vi "LV to ITX Retrieve SM.vi"(0 "File or Folder Path":path=path "C:/", 1 "Data Type":T3=enum."DAT", 2 "DAT header length":i32=11, 5 "offset":i32, 7 "length":i32=1, 11 "error in (no error)":errorcluster) -> (4 "A vs B":cluster{dbl[], dbl[]}[](graph), 6 "C vs D":cluster{dbl[], dbl[]}[](graph), 8 "E":dbl[][](graph), 14 "Notes":string)   [LabVIEW 2019, in "LV-Data.ITX.lvclass"]
uses:
  LV-Data.ITX.lvclass
  <vilib>/Utility/miscctls.llb/LVOffsetAndMultiplierTypeDef.ctl
  Typedefs/Retrieve Data Type.ctl
  LV-Data/Typedefs/Map Variant--map.ctl
  b9190c8c-04b9-4fe6-9890-9f3313ef96ba.vi
  59021a08-4f23-4d52-b62b-93f2ba281558.vi
  LV-Data/LV-Data.lvclass
  <userlib>/LevyLab/Graph Utilities/graph_utilities.lvclass
  <userlib>/LevyLab/Instrument Framework/SMOs/Instrument/Instrument.lvclass
panel:
  out "Current State":string
  in  "Update Graphs":bool
  in  "Read Files":bool
  in  "Initialize Keys":bool
  out "N":T1(array[cluster]) {"N5" format="%#_6p"; "N4" format="%#_6p"; "N3" format="%#_6p"; "N2" format="%#_6p"; "N1" format="%#_6p"}
  in  "keys":T2 {"N5" items=["AI1", "AI10", "AI11", "AI12", "AI2", "AI3", "AI4", "AI5", "AI6", "AI7", "AI8", "AI9", "AO1", "AO10", "AO11", "AO12", "AO2", "AO3", "AO4", "AO5", "AO6", "AO7", "AO8", "AO9", "Magnet", "Magnet Field", "OFF", "Temperature", "Time", "X1", "X10", "X11", "X12", "X2", "X3", "X4", "X5", "X6", "X7", "X8", "X9", "Y1", "Y10", "Y11", "Y12", "Y2", "Y3", "Y4", "Y5", "Y6", "Y7", "Y8", "Y9"]; "N4" items=["AI1", "AI10", "AI11", "AI12", "AI2", "AI3", "AI4", "AI5", "AI6", "AI7", "AI8", "AI9", "AO1", "AO10", "AO11", "AO12", "AO2", "AO3", "AO4", "AO5", "AO6", "AO7", "AO8", "AO9", "Magnet", "Magnet Field", "OFF", "Temperature", "Time", "X1", "X10", "X11", "X12", "X2", "X3", "X4", "X5", "X6", "X7", "X8", "X9", "Y1", "Y10", "Y11", "Y12", "Y2", "Y3", "Y4", "Y5", "Y6", "Y7", "Y8", "Y9"]; "N3" items=["AI1", "AI10", "AI11", "AI12", "AI2", "AI3", "AI4", "AI5", "AI6", "AI7", "AI8", "AI9", "AO1", "AO10", "AO11", "AO12", "AO2", "AO3", "AO4", "AO5", "AO6", "AO7", "AO8", "AO9", "Magnet", "Magnet Field", "OFF", "Temperature", "Time", "X1", "X10", "X11", "X12", "X2", "X3", "X4", "X5", "X6", "X7", "X8", "X9", "Y1", "Y10", "Y11", "Y12", "Y2", "Y3", "Y4", "Y5", "Y6", "Y7", "Y8", "Y9"]; "N2" items=["AI1", "AI10", "AI11", "AI12", "AI2", "AI3", "AI4", "AI5", "AI6", "AI7", "AI8", "AI9", "AO1", "AO10", "AO11", "AO12", "AO2", "AO3", "AO4", "AO5", "AO6", "AO7", "AO8", "AO9", "Magnet", "Magnet Field", "OFF", "Temperature", "Time", "X1", "X10", "X11", "X12", "X2", "X3", "X4", "X5", "X6", "X7", "X8", "X9", "Y1", "Y10", "Y11", "Y12", "Y2", "Y3", "Y4", "Y5", "Y6", "Y7", "Y8", "Y9"]; "N1" items=["AI1", "AI10", "AI11", "AI12", "AI2", "AI3", "AI4", "AI5", "AI6", "AI7", "AI8", "AI9", "AO1", "AO10", "AO11", "AO12", "AO2", "AO3", "AO4", "AO5", "AO6", "AO7", "AO8", "AO9", "Magnet", "Magnet Field", "OFF", "Temperature", "Time", "X1", "X10", "X11", "X12", "X2", "X3", "X4", "X5", "X6", "X7", "X8", "X9", "Y1", "Y10", "Y11", "Y12", "Y2", "Y3", "Y4", "Y5", "Y6", "Y7", "Y8", "Y9"]; "E" items=["AI1", "AI10", "AI11", "AI12", "AI2", "AI3", "AI4", "AI5", "AI6", "AI7", "AI8", "AI9", "AO1", "AO10", "AO11", "AO12", "AO2", "AO3", "AO4", "AO5", "AO6", "AO7", "AO8", "AO9", "Magnet", "Magnet Field", "OFF", "Temperature", "Time", "X1", "X10", "X11", "X12", "X2", "X3", "X4", "X5", "X6", "X7", "X8", "X9", "Y1", "Y10", "Y11", "Y12", "Y2", "Y3", "Y4", "Y5", "Y6", "Y7", "Y8", "Y9"]; "D" items=["AI1", "AI10", "AI11", "AI12", "AI2", "AI3", "AI4", "AI5", "AI6", "AI7", "AI8", "AI9", "AO1", "AO10", "AO11", "AO12", "AO2", "AO3", "AO4", "AO5", "AO6", "AO7", "AO8", "AO9", "Magnet", "Magnet Field", "OFF", "Temperature", "Time", "X1", "X10", "X11", "X12", "X2", "X3", "X4", "X5", "X6", "X7", "X8", "X9", "Y1", "Y10", "Y11", "Y12", "Y2", "Y3", "Y4", "Y5", "Y6", "Y7", "Y8", "Y9"]; "C" items=["AI1", "AI10", "AI11", "AI12", "AI2", "AI3", "AI4", "AI5", "AI6", "AI7", "AI8", "AI9", "AO1", "AO10", "AO11", "AO12", "AO2", "AO3", "AO4", "AO5", "AO6", "AO7", "AO8", "AO9", "Magnet", "Magnet Field", "OFF", "Temperature", "Time", "X1", "X10", "X11", "X12", "X2", "X3", "X4", "X5", "X6", "X7", "X8", "X9", "Y1", "Y10", "Y11", "Y12", "Y2", "Y3", "Y4", "Y5", "Y6", "Y7", "Y8", "Y9"]; "B" items=["AI1", "AI10", "AI11", "AI12", "AI2", "AI3", "AI4", "AI5", "AI6", "AI7", "AI8", "AI9", "AO1", "AO10", "AO11", "AO12", "AO2", "AO3", "AO4", "AO5", "AO6", "AO7", "AO8", "AO9", "Magnet", "Magnet Field", "OFF", "Temperature", "Time", "X1", "X10", "X11", "X12", "X2", "X3", "X4", "X5", "X6", "X7", "X8", "X9", "Y1", "Y10", "Y11", "Y12", "Y2", "Y3", "Y4", "Y5", "Y6", "Y7", "Y8", "Y9"]; "A" items=["AI1", "AI10", "AI11", "AI12", "AI2", "AI3", "AI4", "AI5", "AI6", "AI7", "AI8", "AI9", "AO1", "AO10", "AO11", "AO12", "AO2", "AO3", "AO4", "AO5", "AO6", "AO7", "AO8", "AO9", "Magnet", "Magnet Field", "OFF", "Temperature", "Time", "X1", "X10", "X11", "X12", "X2", "X3", "X4", "X5", "X6", "X7", "X8", "X9", "Y1", "Y10", "Y11", "Y12", "Y2", "Y3", "Y4", "Y5", "Y6", "Y7", "Y8", "Y9"]}
  in  "OK":bool
  in  "D  is time?":bool
  in  "B is time?":bool
  out "time":string[][](table)
  in  "Use Folder Index File?":bool
  in  "Generate Folder Index File?":bool
  in  "Ez name":string="Ez name"
  in  "Ey name":string="Ey name"
  in  "Ex name":string="Ex name"
  in  "C y name":string="C y name"
  in  "D x name":string="D x name"
  in  "A y name":string="A y name"
  in  "B x name":string="B x name"
  out "Index, Wavenames":string[][](table)
  in  "recolor traces?":bool
  in  "Ex":T4={"Offset"=0.0, "Multiplier"=1.0}
  in  "Ey":T4={"Offset"=0.0, "Multiplier"=1.0}
  out "counter":i32
  out "pattern":string="*.dat"
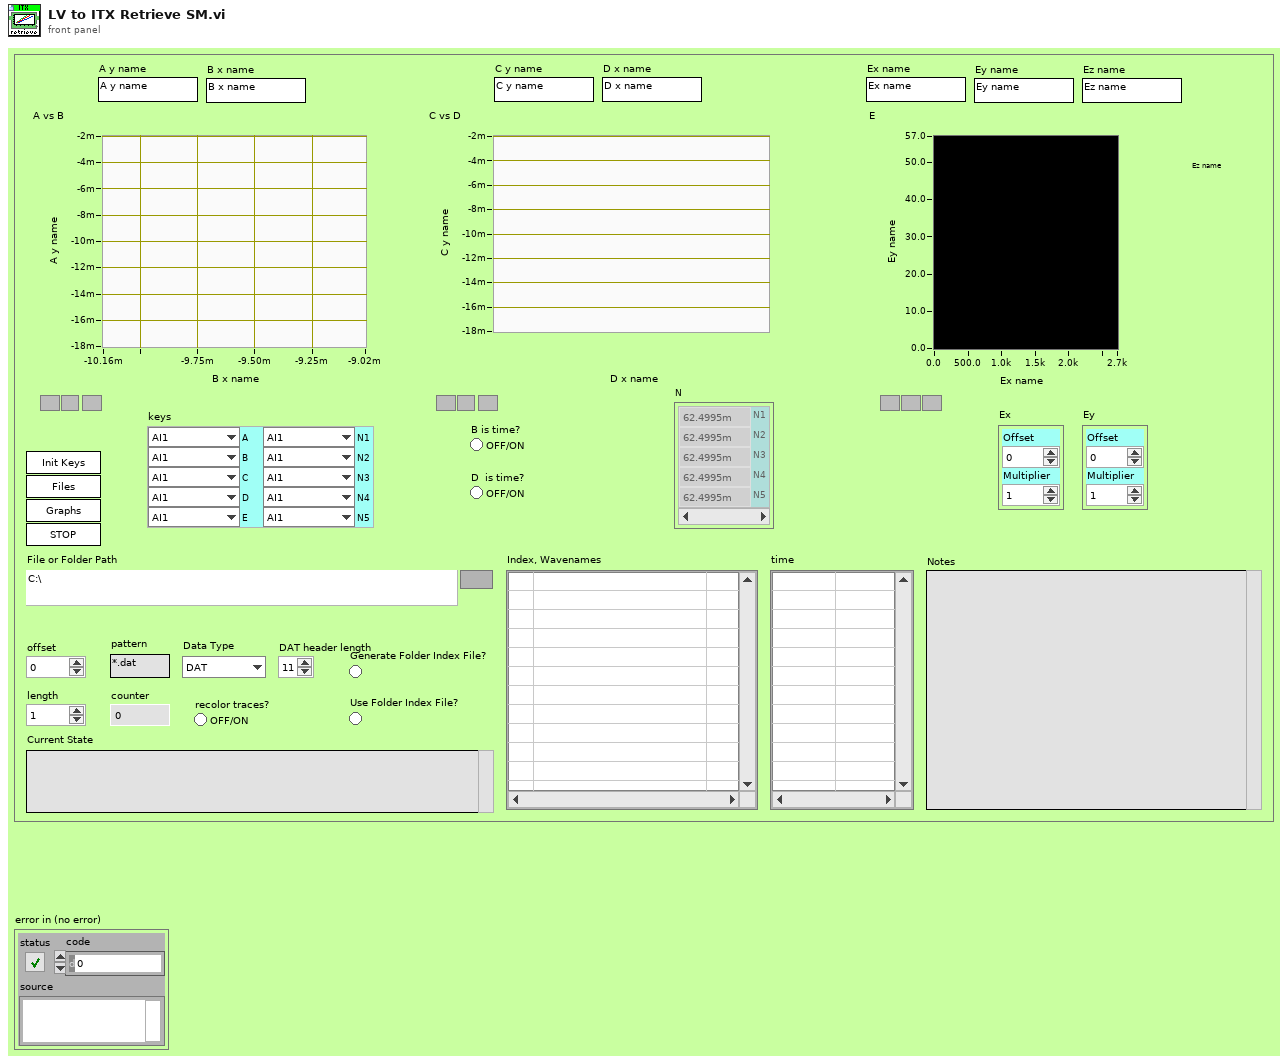
[diagram p1: front panel]
types:
  T1 = cluster{"N1":dbl, "N2":dbl, "N3":dbl, "N4":dbl, "N5":dbl}[]
  T2 = cluster{"A":u16, "B":u16, "C":u16, "D":u16, "E":u16, "N1":u16, "N2":u16, "N3":u16, "N4":u16, "N5":u16}
  T3 = typedef "LV-Data.ITX.lvclass/Retrieve Data Type.ctl" = enum16{"ITX", "ITX w/ 2D", "DAT", "TDMS"}
  T4 = typedef "LVOffsetAndMultiplierTypeDef.ctl" = cluster{"Offset":dbl, "Multiplier":dbl}
  T5 = enum32{"Invalid", "Standard", "Closed", "Hidden", "Minimized", "Maximized"}
  T6 = enum32{"invalid app kind", "Development System", "Run Time System", "Student Edition", "Embedded LabVIEW", "Evaluation", "Custom"}
  T7 = typedef "LV-Data.lvclass/Map Variant--map.ctl" = map{string, variant}
  T8 = cluster{"N1":dbl, "N2":dbl, "N3":dbl, "N4":dbl, "N5":dbl}
  T9 = cluster{"Core":cluster{"Current VI Reference":refnum<vi>, "Close Panel on Exit?":bool}, "Files":path[], "Append Index":i32, "Running Step":i32, "Data Map":T7[], "ring map":map{string, refnum<vi>}, "Wavenames":string[], "A vs B":cluster{dbl[], dbl[]}[], "C vs D":cluster{dbl[], dbl[]}[], "E":dbl[][]}
  T10 = cluster{"Current VI Reference":refnum<vi>, "Close Panel on Exit?":bool}
  T11 = typedef "LV-Data.lvclass/Dictionary--cluster.ctl" = cluster{"key":string, "value":variant}
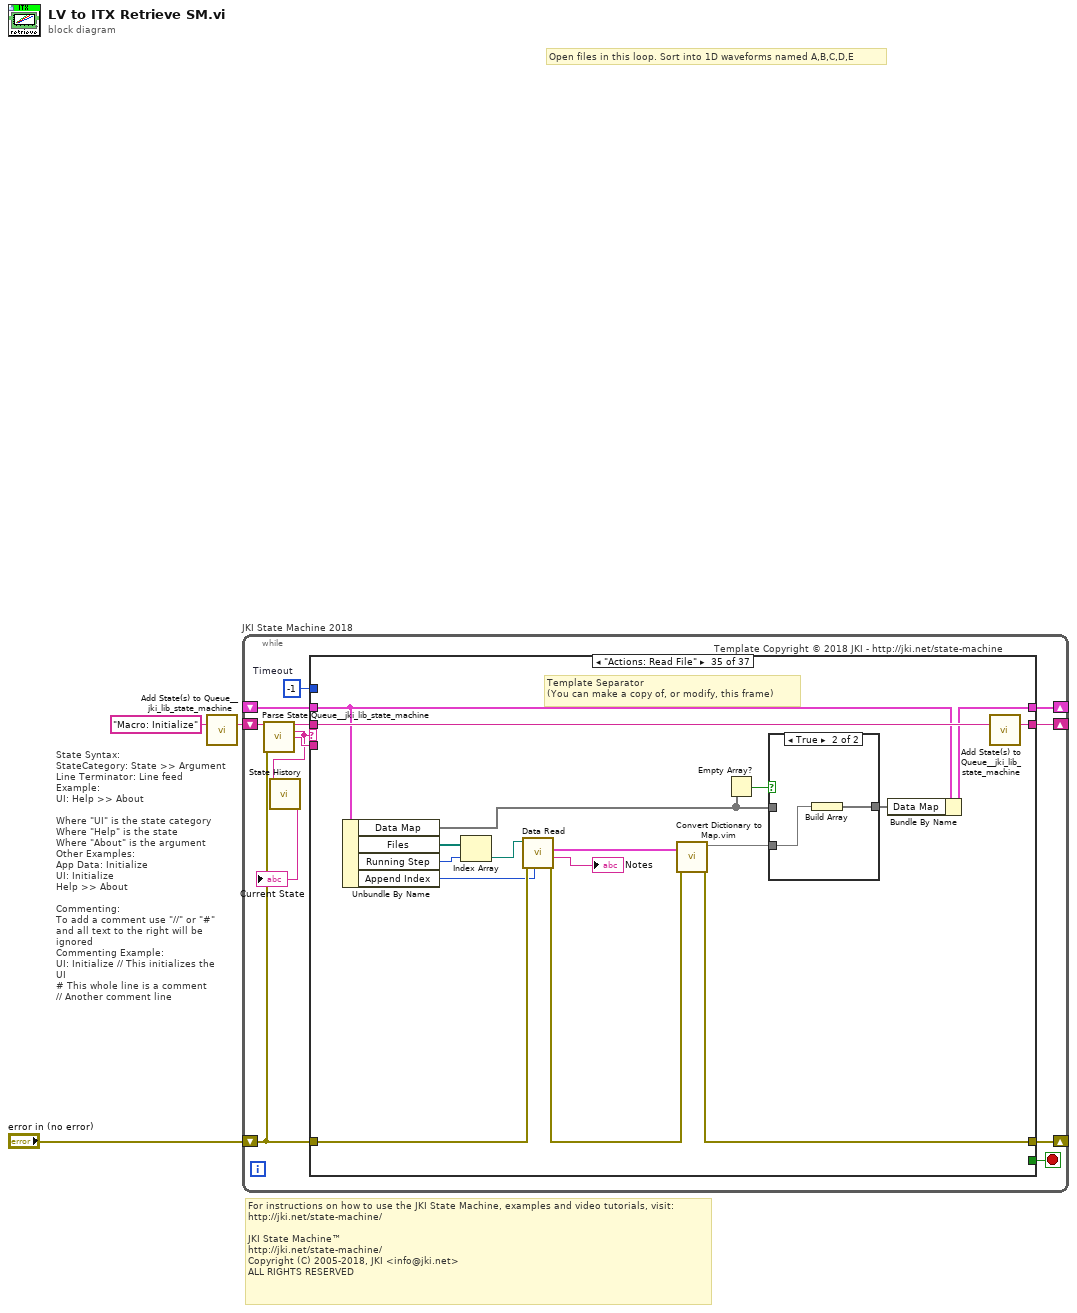
[diagram p0: block diagram]
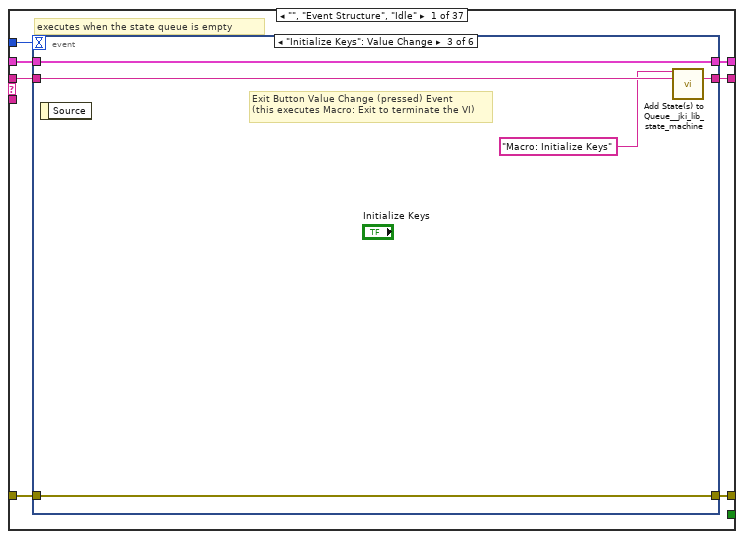
[diagram p2: hidden frame]
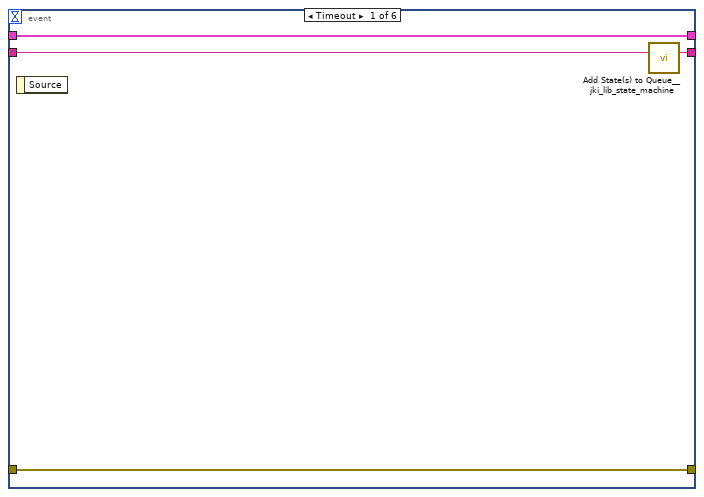
[diagram p3: hidden frame]
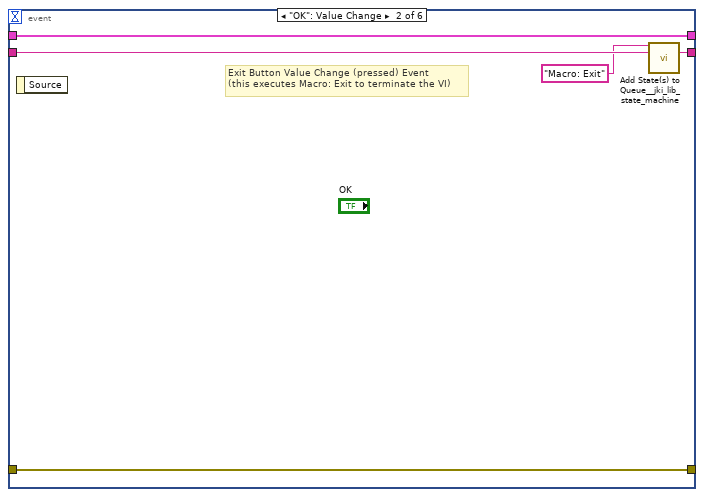
[diagram p4: hidden frame]
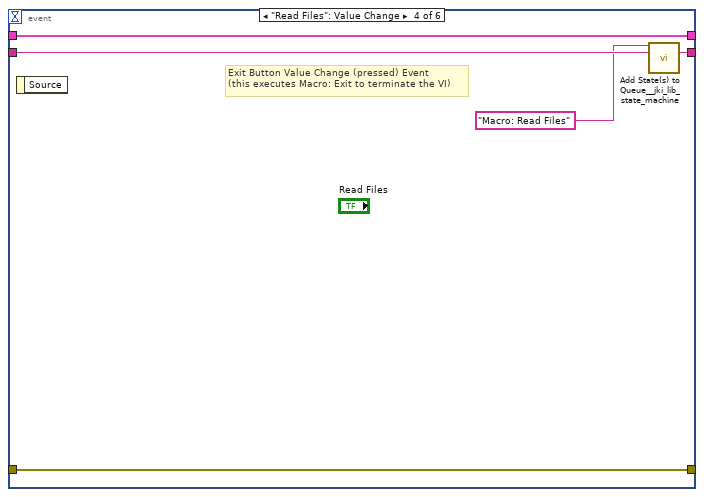
[diagram p5: hidden frame]
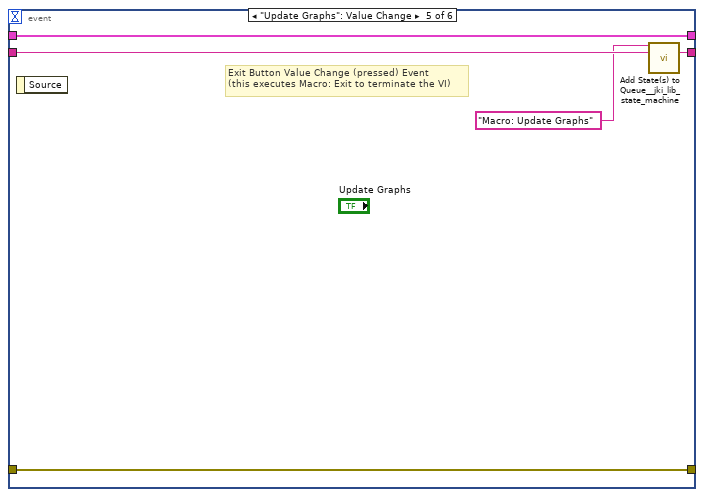
[diagram p6: hidden frame]
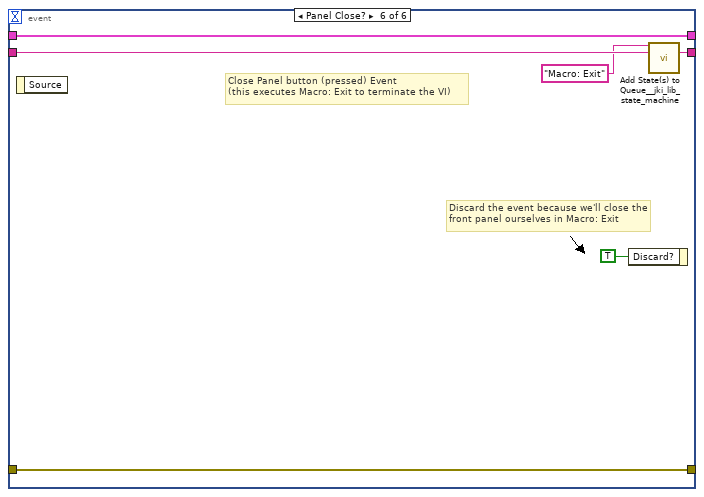
[diagram p7: hidden frame]
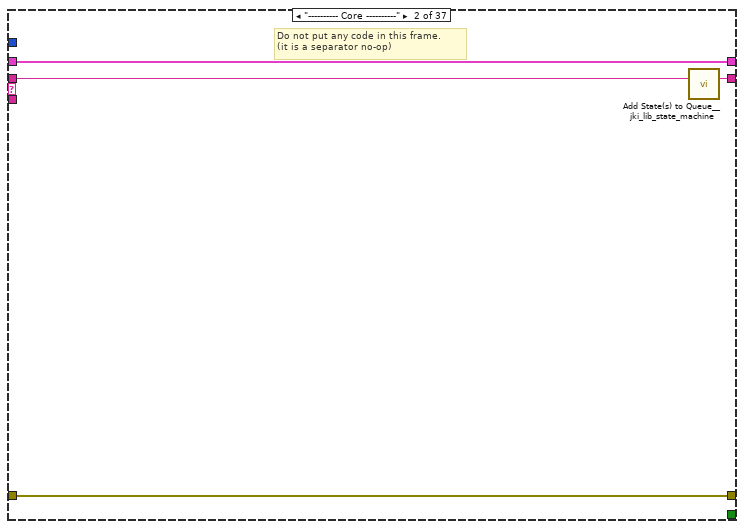
[diagram p8: hidden frame]
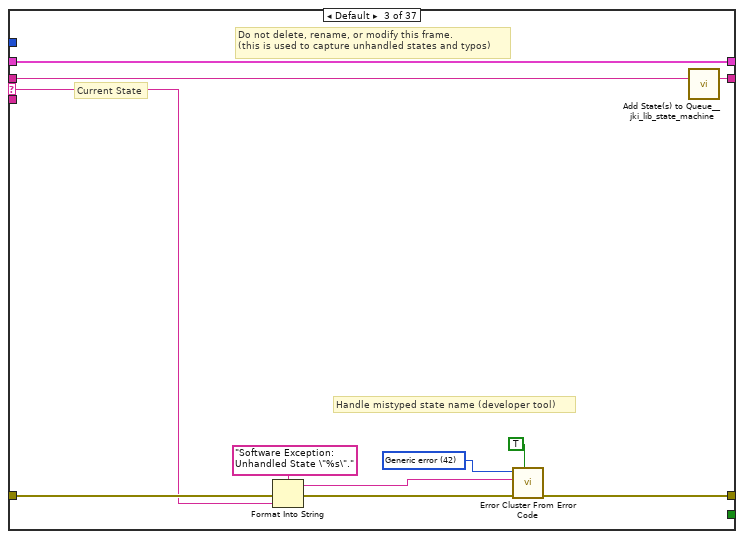
[diagram p9: hidden frame]
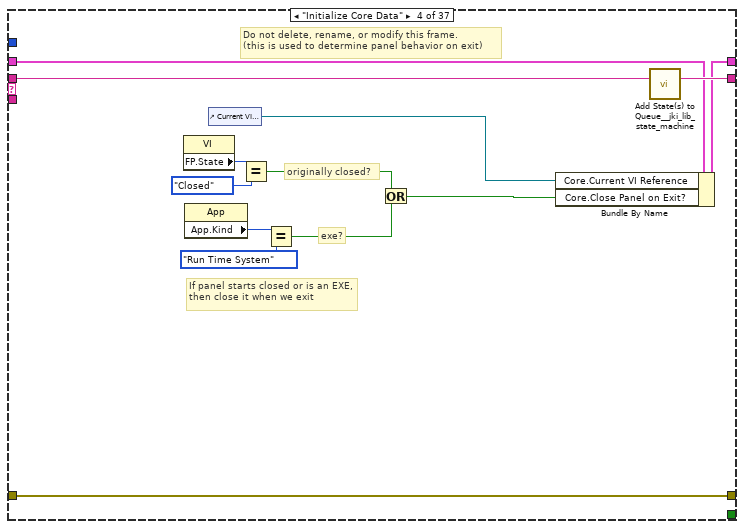
[diagram p10: hidden frame]
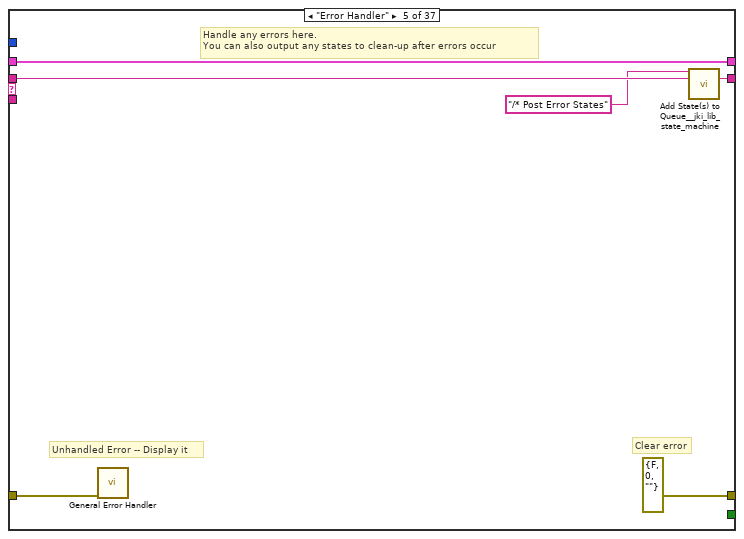
[diagram p11: hidden frame]
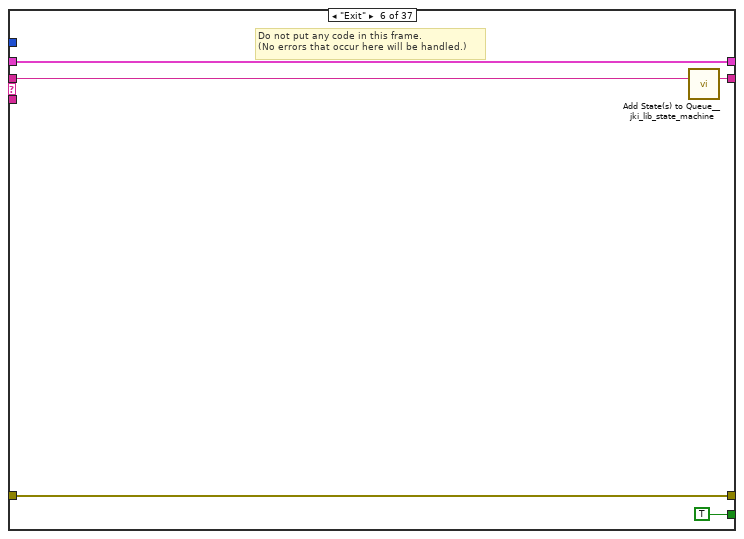
[diagram p12: hidden frame]
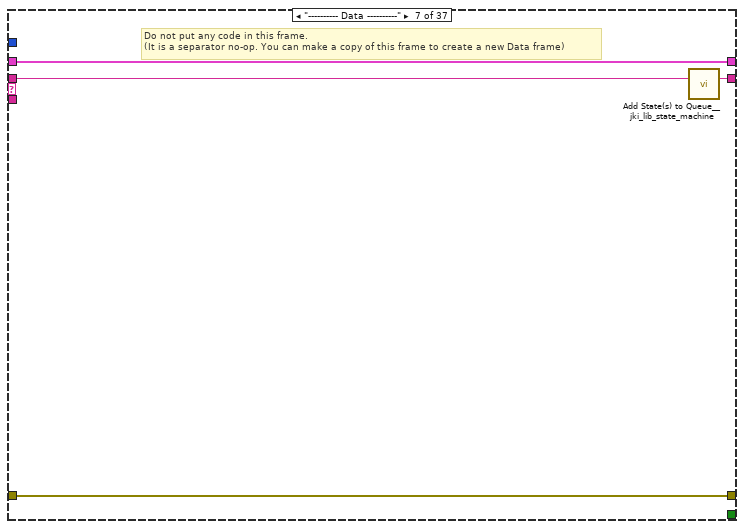
[diagram p13: hidden frame]
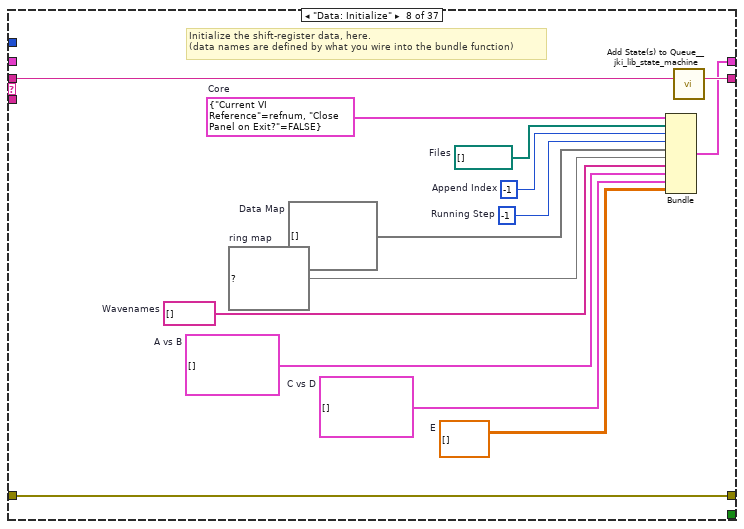
[diagram p14: hidden frame]
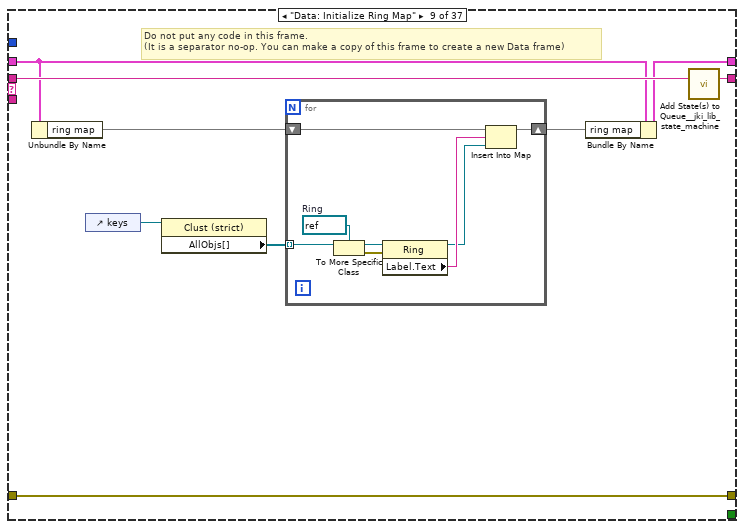
[diagram p15: hidden frame]
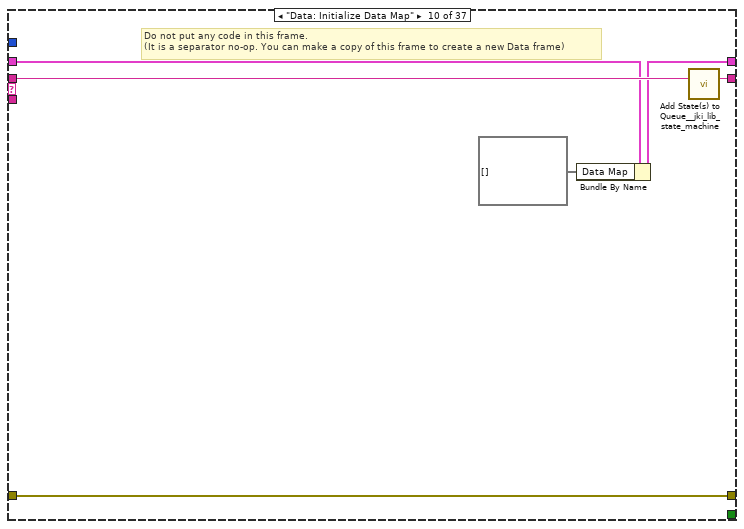
[diagram p16: hidden frame]
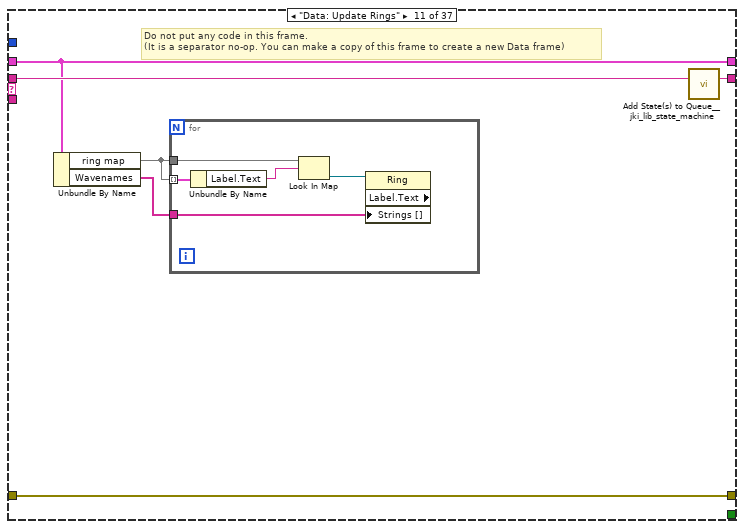
[diagram p17: hidden frame]
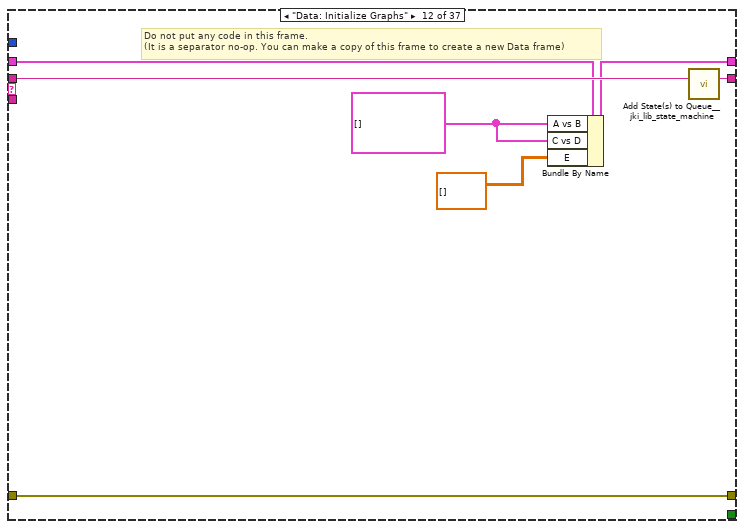
[diagram p18: hidden frame]
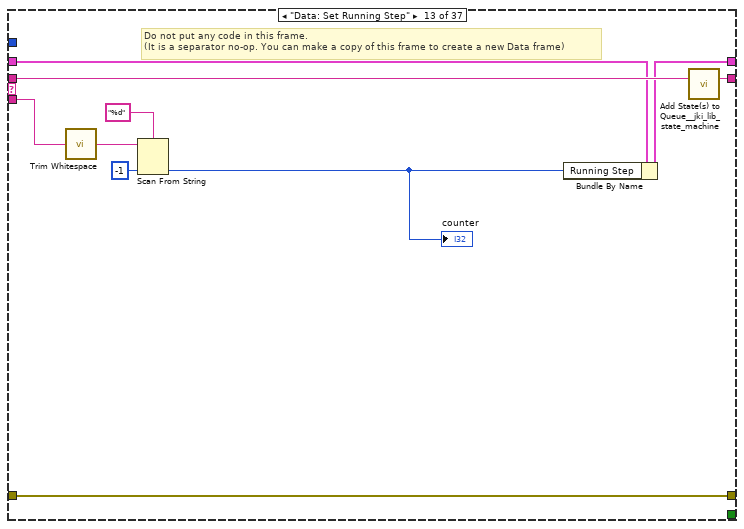
[diagram p19: hidden frame]
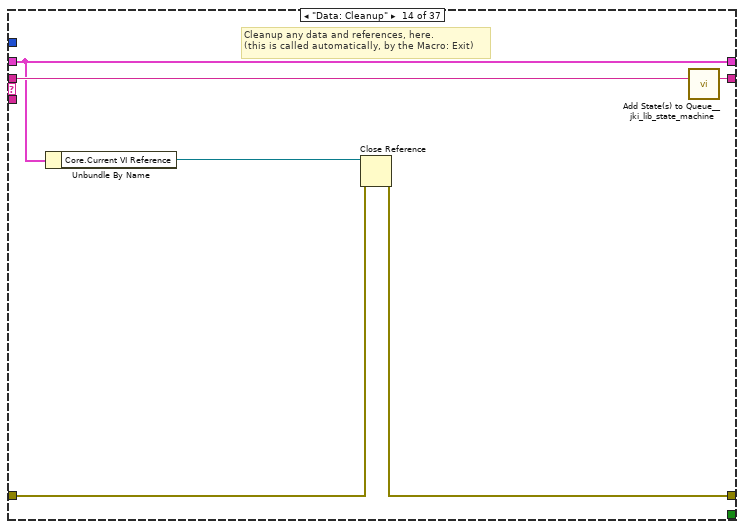
[diagram p20: hidden frame]
diagram:
  # "For instructions on how to use the JKI State Machine, examples and video tutorials, visit:\nhttp://jki.net/state-machine/\n\nJKI State Machine™\nhttp://jki.net/state-machine/\nCopyright (C) 2005-2018, JKI <info@jki.net>\nALL RIGHTS RESERVED"
  # "State Syntax:\nStateCategory: State >> Argument\nLine Terminator: Line feed\nExample:\nUI: Help >> About\n\nWhere \"UI\" is the state category\nWhere \"Help\" is the state\nWhere \"About\" is the argument\nOther Examples:\nApp Data: Initialize\nUI: Initialize\nHelp >> About\n\nCommenting:\nTo add a comment use \"//\" or \"#\" and all text to the right will be ignored\nCommenting Example:\nUI: Initialize // This initializes the UI\n# This whole line is a comment\n// Another comment line"
  # "Open files in this loop. Sort into 1D waveforms named A,B,C,D,E"
  n1 = call <vilib>:"Add State(s) to Queue__jki_lib_state_machine.vi"("State(s) in (\"\")"="Macro: Initialize") -> ("States Out"=w3:string)  [unwired: 14 in]
  n2 = while "JKI State Machine 2018" {
    shift-right: [w9] -> _
    shift-left: _ -> [w8]
    shift-right: [w12] -> _
    shift-left: "error in (no error)" -> [w6]
    shift-right: [w11] -> _
    shift-left: w3 -> [w13]
    stop <- w10 stop-if-true
    w7 = -1  # Timeout
    # "Template Copyright © 2018 JKI - http://jki.net/state-machine"
    n3 = call <vilib>:"Parse State Queue__jki_lib_state_machine.vi"("State Queue"=w13, "Error In (no error)"=w6) -> ("Remaining States"=w15:string, "Current State"=w5:string, "Arguments"=w14:string)  [unwired: 11 in]
    n4 = call <userlib>:"State History.vi"("Current State"=w5) -> ("History"=→"Current State":string)  [unwired: 10 in]
    n5 = case shown="\"Actions: Read File\"" w5 {
      selector: w5 -> [_ _ w57 _ _ _ _ _ _ _ _ _ _ _ _ _ _ _ _ _ _ _ _ _ _ _ _ _ _ _ _ _ _ _ _ _ _]
      tunnel: w15 -> [w22 w56 w61 w80 w86 w91 w95 w109 w118 w132 w138 w150 w160 w166 w170 w176 w182 w194 w200 w228 w235 w304 w309 w314 w329 w334 w339 w344 w349 w359 w363 w377 w424 w446 w465 w499 w520]
      tunnel: w14 -> [_ _ _ _ _ _ _ _ _ _ _ _ w155 _ _ _ w177 _ _ _ w229 _ _ _ w319 _ _ _ _ _ _ _ _ _ _ _ _]
      tunnel: w8 -> [w20 w53 w59 w73 w83 w89 w92 _ w110 w128 w135 w146 w156 w161 w167 w174 w180 w191 w196 w225 w231 w301 w306 w311 w326 w331 w336 w341 w346 w356 w360 w366 w419 w439 w454 w471 w517]
      tunnel: [w19 w54 w63 w77 errorcluster {"status"=FALSE, "code"=0, "source"=""} ("error out") w88 w93 w106 w116 w130 w136 w148 w158 w162 w168 w172 w178 w192 w198 w226 w232 w302 w307 w312 w327 w332 w337 w342 w347 w357 w361 w370 w422 w442 w456 w497 w518] -> w12
      tunnel: w6 -> [w18 w54 w62 w77 w82 w88 w93 w106 w116 w130 w136 w148 w158 w163 w168 w171 w179 w192 w198 w226 w233 w302 w307 w312 w327 w332 w337 w342 w347 w357 w361 w369 w422 w441 w461 w497 w518]
      tunnel: [w21 w55 w60 w79 w85 w90 w94 w108 w117 w131 w137 w149 w159 w165 w169 w175 w181 w193 w199 w227 w234 w303 w308 w313 w328 w333 w338 w343 w348 w358 w362 w376 w423 w445 w464 w498 w519] -> w11
      tunnel: [_ _ _ _ _ TRUE _ _ _ _ _ _ _ _ _ _ _ _ _ _ _ _ _ _ _ _ _ _ _ _ _ _ _ _ _ _ _] -> w10
      tunnel: [w17 w53 w59 w78 w83 w89 w92 w107 w111 w129 w135 w147 w157 w161 w167 w174 w180 w191 w196 w225 w231 w301 w306 w311 w326 w331 w336 w341 w346 w356 w360 w367 w420 w440 w455 w472 w517] -> w9
      tunnel: w7 -> [w16 _ _ _ _ _ _ _ _ _ _ _ _ _ _ _ _ _ _ _ _ _ _ _ _ _ _ _ _ _ _ _ _ _ _ _ _]
      frame "", "Event Structure", "Idle" {
        # "executes when the state queue is empty"
        n6 = event shown="[2] \"Initialize Keys\": Value Change" {
          selector: _ -> [_ _ _ _ _ _]
          dyn-events: _ -> [_ _ _ _ _ _]
          timeout: w16 -> [_ _ _ _ _ _]
          tunnel: w22 -> [w26 w31 w36 w41 w46 w52]
          tunnel: [w25 w30 w35 w40 w45 w51] -> w21
          tunnel: w20 -> [w23 w28 w33 w38 w43 w49]
          tunnel: [w24 w29 w34 w39 w44 w50] -> w19
          tunnel: w18 -> [w24 w29 w34 w39 w44 w50]
          tunnel: [w23 w28 w33 w38 w43 w49] -> w17
          event Timeout {
            n7 = event-data() -> ()  [unwired: 1 in, 1 out]
            n8 = call <vilib>:"Add State(s) to Queue__jki_lib_state_machine.vi"("State(s) in (\"\")"=w26) -> ("States Out"=w25:string)  [unwired: 14 in]
          }
          event "OK": Value Change {
            # "Exit Button Value Change (pressed) Event\n(this executes Macro: Exit to terminate the VI)"
            n9 = event-data() -> ()  [unwired: 1 in, 1 out]
            n10 = call <vilib>:"Add State(s) to Queue__jki_lib_state_machine.vi"("State(s) in Front (\"\")"="Macro: Exit", "State(s) in (\"\")"=w31) -> ("States Out"=w30:string)  [unwired: 13 in]
          }
          event "Initialize Keys": Value Change {
            # "Exit Button Value Change (pressed) Event\n(this executes Macro: Exit to terminate the VI)"
            n11 = event-data() -> ()  [unwired: 1 in, 1 out]
            n12 = call <vilib>:"Add State(s) to Queue__jki_lib_state_machine.vi"("State(s) in Front (\"\")"="Macro: Initialize Keys", "State(s) in (\"\")"=w36) -> ("States Out"=w35:string)  [unwired: 13 in]
          }
          event "Read Files": Value Change {
            # "Exit Button Value Change (pressed) Event\n(this executes Macro: Exit to terminate the VI)"
            n13 = event-data() -> ()  [unwired: 1 in, 1 out]
            n14 = call <vilib>:"Add State(s) to Queue__jki_lib_state_machine.vi"("State(s) in Front (\"\")"="Macro: Read Files", "State(s) in (\"\")"=w41) -> ("States Out"=w40:string)  [unwired: 13 in]
          }
          event "Update Graphs": Value Change {
            # "Exit Button Value Change (pressed) Event\n(this executes Macro: Exit to terminate the VI)"
            n15 = event-data() -> ()  [unwired: 1 in, 1 out]
            n16 = call <vilib>:"Add State(s) to Queue__jki_lib_state_machine.vi"("State(s) in Front (\"\")"="Macro: Update Graphs", "State(s) in (\"\")"=w46) -> ("States Out"=w45:string)  [unwired: 13 in]
          }
          event Panel Close? {
            # "Discard the event because we'll close the front panel ourselves in Macro: Exit"
            # "Close Panel button (pressed) Event\n(this executes Macro: Exit to terminate the VI)"
            n17 = event-data() -> ()  [unwired: 1 in, 1 out]
            n18 = event-data("Discard?"=TRUE) -> ()  [unwired: 1 in, 1 out]
            n19 = call <vilib>:"Add State(s) to Queue__jki_lib_state_machine.vi"("State(s) in Front (\"\")"="Macro: Exit", "State(s) in (\"\")"=w52) -> ("States Out"=w51:string)  [unwired: 13 in]
          }
        }
      }
      frame "---------- Core ----------" {
        # "Do not put any code in this frame.\n(it is a separator no-op)"
        n20 = call <vilib>:"Add State(s) to Queue__jki_lib_state_machine.vi"("State(s) in (\"\")"=w56) -> ("States Out"=w55:string)  [unwired: 14 in]
      }
      frame Default {
        w66 = 42 items=["No error", "Argument error", "Memory is full", "Out of zone", "End of file", "File already open", "Generic file I/O error", "File not found", "File permission error", "Disk is full", "Duplicate path", "Too many files open", "System feature not enabled", "Resource file not found", "Cannot add resource", "Resource not found", "Image not found", "Image memory error", "Pen does not exist", "Config type invalid", "Config token not found", "Config parse error", "Config memory error", "Bad external code format", "Bad external code offset", "External code not present", "Null window", "Destroy window error", "Null menu", "Print aborted", "Bad print record", "Print driver error", "Windows error during printing", "Memory error during printing", "Print dialog error", "Generic print error", "Invalid device refnum", "Device not found", "Device parameter error", "Device unit error", "Cannot open device", "Device call aborted", "Generic error", "Cancelled by user", "Object ID too low", "Object ID too high", "Object not in heap", "Unknown heap", "Unknown object (invalid DefProc)", "Unknown object (DefProc not in table)", "Message out of range", "Invalid (null) method", "Unknown message", "Manager call not supported", "Bad address", "Network operation in progress", "Network operation timed out", "Connection is busy", "Network attribute not supported", "Network error", "Address in use", "System out of memory", "Connection aborted", "Connection refused", "Not connected", "Already connected", "Connection closed", "Initialization error (interapplication manager)", "Bad occurrence", "Wait on unbound occurrence handler", "Occurrence queue overflow", "Datalog type conflict", "Unused", "Unrecognized type (interapplication manager)", "Memory corrupt", "Failed to make temporary DLL", "Old CIN version", "Drag socket not found", "Failed to load drop-object", "Failed to register OLE object", "Failed to release OLE object", "Format specifier type mismatch", "Unknown format specifier", "Too few format specifiers", "Too many format specifiers", "Scan failed", "Newer CIN version", "Error converting to variant", "Runtime menu error", "Password tampered", "Variant attribute not found", "Incompatible variant data type", "Event data is not available", "Event Store is not present", "Occurrence is not found", "Event Queue is not created", "Event info is not available", "Refnum passed is NULL", "Error retrieving Class GUID", "Error retrieving CoClass GUID", "Error retrieving TypeLib GUID.", "Bad built application magic bytes.", "Specific driver is different from the specific driver associated with the Logical Name.", "There is no session opened to the class driver.", "Max Error", "MAX - Error with config objects", "MAX - Error loading configuration", "MAX - Group not supported"]
        # "Current State"
        # "Do not delete, rename, or modify this frame.\n(this is used to capture unhandled states and typos)"
        # "Handle mistyped state name (developer tool)"
        n21 = Format Into String(format string="Software Exception: Unhandled State \"%s\"." ("message"), error in=w62, w57) -> (resulting string=w65:string, error out=w64:errorcluster)  [unwired: 1 in]
        n22 = call <vilib>:"Error Cluster From Error Code.vi"("show call chain? (False)"=TRUE, "error in (no error)"=w64, "error message (\"\")"=w65, "error code (0)"=w66) -> ("error out"=w63:errorcluster)  [unwired: 5 in]
        n23 = call <vilib>:"Add State(s) to Queue__jki_lib_state_machine.vi"("State(s) in (\"\")"=w61) -> ("States Out"=w60:string)  [unwired: 14 in]
      }
      frame "Initialize Core Data" {
        # "Do not delete, rename, or modify this frame.\n(this is used to determine panel behavior on exit)"
        # "originally closed?"
        # "exe?"
        # "If panel starts closed or is an EXE, then close it when we exit"
        n24 = property class="VI"() -> ("FP.State"=w70:T5)  [unwired: 2 in, 2 out]
        n25 = property class="App"() -> ("App.Kind"=w76:T6)  [unwired: 2 in, 2 out]
        n26 = control-ref of="Current VI Reference"() -> (w71:refnum<vi>)
        n27 = Equal?(x=w70, y=T5."Closed" ("Front Panel Window:State")) -> (x = y?=w68:bool)
        n28 = Equal?(x=w76, y=T6."Run Time System" ("Application:Kind")) -> (x = y?=w74:bool)
        n29 = Or(x=w68, y=w74) -> (x .or. y?=w72:bool)
        n30 = Bundle By Name(cluster=w73, "Core.Current VI Reference"=w71, "Core.Close Panel on Exit?"=w72) -> (w78:T9)
        n31 = call <vilib>:"Add State(s) to Queue__jki_lib_state_machine.vi"("State(s) in (\"\")"=w80) -> ("States Out"=w79:string)  [unwired: 14 in]
      }
      frame "Error Handler" {
        # "Unhandled Error -- Display it"
        # "Handle any errors here.\nYou can also output any states to clean-up after errors occur"
        # "Clear error"
        n32 = call <vilib>:"General Error Handler.vi"("error in (no error)"=w82) -> ()  [unwired: 10 in, 5 out]
        n33 = call <vilib>:"Add State(s) to Queue__jki_lib_state_machine.vi"("State(s) in Front (\"\")"="/* Post Error States", "State(s) in (\"\")"=w86) -> ("States Out"=w85:string)  [unwired: 13 in]
      }
      frame "Exit" {
        # "Do not put any code in this frame.\n(No errors that occur here will be handled.)"
        n34 = call <vilib>:"Add State(s) to Queue__jki_lib_state_machine.vi"("State(s) in (\"\")"=w91) -> ("States Out"=w90:string)  [unwired: 14 in]
      }
      frame "---------- Data ----------" {
        # "Do not put any code in this frame.\n(It is a separator no-op. You can make a copy of this frame to create a new Data frame)"
        n35 = call <vilib>:"Add State(s) to Queue__jki_lib_state_machine.vi"("State(s) in (\"\")"=w95) -> ("States Out"=w94:string)  [unwired: 14 in]
      }
      frame "Data: Initialize" {
        w96 = dbl[][] []  # E
        w97 = cluster{dbl[], dbl[]}[] []  # C vs D
        w98 = cluster{dbl[], dbl[]}[] []  # A vs B
        w99 = string[] []  # Wavenames
        w100 = map{string, refnum<vi>} {}  # ring map
        w101 = T7[] []  # Data Map
        w102 = -1  # Running Step
        w103 = -1  # Append Index
        w104 = path[] []  # Files
        w105 = T10 {"Current VI Reference"=refnum, "Close Panel on Exit?"=FALSE}  # Core
        # "Initialize the shift-register data, here.\n(data names are defined by what you wire into the bundle function)"
        n36 = Bundle("Core"=w105, "Files"=w104, "Append Index"=w103, "Running Step"=w102, "Data Map"=w101, "ring map"=w100, "Wavenames"=w99, "A vs B"=w98, "C vs D"=w97, "E"=w96) -> (w107:T9)  [unwired: 1 in]
        n37 = call <vilib>:"Add State(s) to Queue__jki_lib_state_machine.vi"("State(s) in (\"\")"=w109) -> ("States Out"=w108:string)  [unwired: 14 in]
      }
      frame "Data: Initialize Ring Map" {
        # "Do not put any code in this frame.\n(It is a separator no-op. You can make a copy of this frame to create a new Data frame)"
        n38 = Unbundle By Name(w110) -> ("ring map"=w113:map{string, refnum<vi>})
        n39 = control-ref of="keys"() -> (w115:refnum<vi>)
        n40 = property class="Clust (strict)"(reference=w115) -> ("AllObjs[]"=w114:refnum<vi>[])  [unwired: 1 in, 2 out]
        n41 = for {
          tunnel: w114 -> [w125] mode=indexing
          shift-right: [w122] -> w112
          shift-left: w113 -> [w121]
          w126 = refnum<vi> refnum  # Ring
          n42 = To More Specific Class(target class=w126, reference=w125) -> (specific class reference=w124:refnum<vi>, error out=w120:errorcluster)  [unwired: 1 in]
          n43 = property class="Ring"(reference=w124, error in=w120) -> (reference out=w119:refnum<vi>, "Label.Text"=w123:string)  [unwired: 1 out]
          n44 = Insert Into Map(map in=w121, key=w123, value=w119) -> (map out=w122:map{string, refnum<vi>})  [unwired: 2 out]
        }
        n45 = Bundle By Name(cluster=w110, "ring map"=w112) -> (w111:T9)
        n46 = call <vilib>:"Add State(s) to Queue__jki_lib_state_machine.vi"("State(s) in (\"\")"=w118) -> ("States Out"=w117:string)  [unwired: 14 in]
      }
      frame "Data: Initialize Data Map" {
        # "Do not put any code in this frame.\n(It is a separator no-op. You can make a copy of this frame to create a new Data frame)"
        n47 = Bundle By Name(cluster=w128, "Data Map"=T7[] []) -> (w129:T9)
        n48 = call <vilib>:"Add State(s) to Queue__jki_lib_state_machine.vi"("State(s) in (\"\")"=w132) -> ("States Out"=w131:string)  [unwired: 14 in]
      }
      frame "Data: Update Rings" {
        # "Do not put any code in this frame.\n(It is a separator no-op. You can make a copy of this frame to create a new Data frame)"
        n49 = Unbundle By Name(w135) -> ("ring map"=w134:map{string, refnum<vi>}, "Wavenames"=w133:string[])
        n50 = for {
          tunnel: w134 -> [w143] mode=indexing
          tunnel: w134 -> [w142]
          tunnel: w133 -> [w139]
          n51 = Unbundle By Name(w143) -> ("Label.Text"=w141:string)
          n52 = Look In Map(map=w142, key=w141) -> (value=w140:refnum<vi>)  [unwired: 1 in, 1 out]
          n53 = property class="Ring" props=["Label", "Text", "Strings []"](reference=w140, "Strings []"=w139) -> ()  [unwired: 1 in, 3 out]
        }
        n54 = call <vilib>:"Add State(s) to Queue__jki_lib_state_machine.vi"("State(s) in (\"\")"=w138) -> ("States Out"=w137:string)  [unwired: 14 in]
      }
      frame "Data: Initialize Graphs" {
        w145 = cluster{dbl[], dbl[]}[] [] ("A vs B")
        # "Do not put any code in this frame.\n(It is a separator no-op. You can make a copy of this frame to create a new Data frame)"
        n55 = Bundle By Name(cluster=w146, "A vs B"=w145, "C vs D"=w145, "E"=dbl[][] []) -> (w147:T9)
        n56 = call <vilib>:"Add State(s) to Queue__jki_lib_state_machine.vi"("State(s) in (\"\")"=w150) -> ("States Out"=w149:string)  [unwired: 14 in]
      }
      frame "Data: Set Running Step" {
        # "Do not put any code in this frame.\n(It is a separator no-op. You can make a copy of this frame to create a new Data frame)"
        n57 = call <vilib>:"Trim Whitespace.vi"("string"=w155) -> ("trimmed string"=w154:string)  [unwired: 1 in]
        n58 = Scan From String(format string="%d", input string=w154, default 1=-1 ("default value 1")) -> (output 1=w151:i32)  [unwired: 2 in, 3 out]
        "counter" <- w151
        n59 = Bundle By Name(cluster=w156, "Running Step"=w151) -> (w157:T9)
        n60 = call <vilib>:"Add State(s) to Queue__jki_lib_state_machine.vi"("State(s) in (\"\")"=w160) -> ("States Out"=w159:string)  [unwired: 14 in]
      }
      frame "Data: Cleanup" {
        # "Cleanup any data and references, here.\n(this is called automatically, by the Macro: Exit)"
        n61 = Unbundle By Name(w161) -> ("Core.Current VI Reference"=w164:refnum<vi>)
        n62 = Close Reference(reference=w164, error in (no error)=w163) -> (error out=w162:errorcluster)
        n63 = call <vilib>:"Add State(s) to Queue__jki_lib_state_machine.vi"("State(s) in (\"\")"=w166) -> ("States Out"=w165:string)  [unwired: 14 in]
      }
      frame "---------- UI ----------" {
        # "Do not put any code in this frame.\n(It is a separator no-op. You can make a copy of this frame to create a new UI frame)"
        n64 = call <vilib>:"Add State(s) to Queue__jki_lib_state_machine.vi"("State(s) in (\"\")"=w170) -> ("States Out"=w169:string)  [unwired: 14 in]
      }
      frame "UI: Initialize" {
        # "Initialize the User Interface, here.\n(this is called automatically, by the Macro: Init)"
        n65 = call <userlib>:"Fit VI window to Largest Dec__ogtk.vi"("error in (no error)"=w171, "border spacing (2 px)"=0) -> ("error out"=w172:errorcluster)  [unwired: 4 in, 1 out]
        n66 = call <vilib>:"Add State(s) to Queue__jki_lib_state_machine.vi"("State(s) in (\"\")"=w176) -> ("States Out"=w175:string)  [unwired: 14 in]
      }
      frame "UI: Cursor Set" {
        # "Argument"
        # "Set and Unset Cursor Busy.\n(Usage: \"UI: Cursor Set >> Busy|Idle\")"
        n67 = case shown="\"Idle\", Default" w177 {
          tunnel: w179 -> [w184 w186]
          tunnel: [w183 w185] -> w178
          frame "Idle", Default {
            n68 = call <vilib>:"Unset Busy.vi"("error in (no error)"=w184) -> ("error out"=w183:errorcluster)  [unwired: 10 in]
          }
          frame "Busy" {
            n69 = call <vilib>:"Set Busy.vi"("error in (no error)"=w186) -> ("error out"=w185:errorcluster)  [unwired: 9 in, 1 out]
          }
        }
        n70 = call <vilib>:"Add State(s) to Queue__jki_lib_state_machine.vi"("State(s) in (\"\")"=w182) -> ("States Out"=w181:string)  [unwired: 14 in]
      }
      frame "UI: Update Graphs" {
        # "Do not put any code in this frame.\n(It is a separator no-op. You can make a copy of this frame to create a new UI frame)"
        n71 = Unbundle By Name(w191) -> ("A vs B"=→"A vs B":cluster{dbl[], dbl[]}[], "C vs D"=→"C vs D":cluster{dbl[], dbl[]}[], "E"=w188:dbl[][])
        n72 = Transpose 2D Array(2D array=w188) -> (transposed array=→"E":dbl[][])
        n73 = call <vilib>:"Add State(s) to Queue__jki_lib_state_machine.vi"("State(s) in (\"\")"=w194) -> ("States Out"=w193:string)  [unwired: 14 in]
      }
      frame "UI: Recolor Graphs" {
        # "Template Separator\n(You can make a copy of, or modify, this frame)"
        n74 = Unbundle By Name(w196) -> ("A vs B"=w195:cluster{dbl[], dbl[]}[])
        n75 = case shown="True" "recolor traces?" {
          tunnel: w195 -> [_ w201]
          frame False {
          }
          frame True {
            n76 = Array Size(array=w201) -> (size(s)=w204:i32)
            n77 = call <userlib>:"Choose Color Table.vi"() -> ("Color Table"=w202:u32[])  [unwired: 8 in, 3 out]
            n78 = call <userlib>:"Choose Color Table.vi"("Size (256)"=w204) -> ("Color Table"=w203:u32[])  [unwired: 7 in, 3 out]
            n79 = for {
              tunnel: w203 -> [w205] mode=indexing
              i -> [w206]
              n80 = property on="A vs B" class="XYGraph (strict)"("Active Plot"=w206, "Plot.Plot Color"=w205) -> (error out=w207:errorcluster)  [unwired: 2 in, 1 out]
              n81 = property on="C vs D" class="XYGraph (strict)"(error in=w207, "Active Plot"=w206, "Plot.Plot Color"=w205, "Plot.Fill/Pt. Color"=w205) -> ()  [unwired: 1 in, 2 out]
            }
            n82 = property on="E" class="IntGraph (strict)"("Color Table"=w202) -> ()  [unwired: 2 in, 2 out]
          }
        }
        n83 = call <vilib>:"Add State(s) to Queue__jki_lib_state_machine.vi"("State(s) in (\"\")"=w200) -> ("States Out"=w199:string)  [unwired: 14 in]
      }
      frame "UI: Graph Labels" {
        # "Do not put any code in this frame.\n(It is a separator no-op. You can make a copy of this frame to create a new UI frame)"
        n84 = property on="E" class="IntGraph (strict)"("XScale.Ofst&Mult"="Ex", "YScale.Ofst&Mult"="Ey") -> ()  [unwired: 2 in, 2 out]
        n85 = property on="E" class="IntGraph (strict)"("XScale.NameLbl.Text"="Ex name", "YScale.NameLbl.Text"="Ey name", "ZScale.NameLbl.Text"="Ez name") -> ()  [unwired: 2 in, 2 out]
        n86 = Select(t=7.0, s="D  is time?", f=8.0) -> (s? t:f=w222:dbl)
        n87 = Select(t=7.0, s="B is time?", f=8.0) -> (s? t:f=w221:dbl)
        n88 = property on="A vs B" class="XYGraph (strict)"("XScale.Format"=w221, "XScale.NameLbl.Text"="B x name", "YScale.NameLbl.Text"="A y name") -> ()  [unwired: 2 in, 2 out]
        n89 = property on="C vs D" class="XYGraph (strict)"("XScale.Format"=w222, "XScale.NameLbl.Text"="D x name", "YScale.NameLbl.Text"="C y name") -> ()  [unwired: 2 in, 2 out]
        n90 = call <vilib>:"Add State(s) to Queue__jki_lib_state_machine.vi"("State(s) in (\"\")"=w228) -> ("States Out"=w227:string)  [unwired: 14 in]
      }
      frame "UI: Front Panel State" {
        # "Argument"
        # "Set Front Panel Open or Closed\n(Usage: \"UI: Front Panel State >> Open|Close\")"
        n91 = Unbundle By Name(w231) -> ("Core.Current VI Reference"=w230:refnum<vi>)
        n92 = case shown="\"Minimize\", \"Minimized\"" w229 {
          tunnel: w233 -> [w241 w256 w267 w280 w293]
          tunnel: [w243 w257 w269 w282 w295] -> w232
          tunnel: w230 -> [w242 w254 w268 w281 w294]
          frame "Open", "Standard", Default {
            w236 = T5."Standard" ("State")
            n93 = property class="VI"(reference=w242, error in=w241) -> (reference out=w239:refnum<vi>, error out=w240:errorcluster, "FP.State"=w238:T5)
            n94 = Not Equal?(x=w238, y=w236) -> (x != y?=w237:bool)
            n95 = case shown="True" w237 {
              tunnel: [w247 w249] -> w243
              tunnel: w240 -> [w246 w249]
              tunnel: w239 -> [w245 _]
              tunnel: w236 -> [w244 _]
              frame True {
                n96 = invoke class="VI" method="FP.Open"(reference=w245, error in=w246, "Activate"=TRUE, "State"=w244) -> (error out=w247:errorcluster)  [unwired: 1 in, 4 out]
              }
              frame False {
              }
            }
          }
          frame "Close", "Closed" {
            n97 = property class="VI"(reference=w254, error in=w256) -> (reference out=w253:refnum<vi>, error out=w255:errorcluster, "FP.State"=w251:T5)
            n98 = Not Equal?(x=w251, y=T5."Closed" ("Front Panel Window:State")) -> (x != y?=w250:bool)
            n99 = case shown="True" w250 {
              tunnel: [w258 w261] -> w257
              tunnel: w255 -> [w258 w260]
              tunnel: w253 -> [_ w259]
              frame False {
              }
              frame True {
                n100 = invoke class="VI" method="FP.Close"(reference=w259, error in=w260) -> (error out=w261:errorcluster)  [unwired: 1 in, 2 out]
              }
            }
          }
          frame "Hidden", "Hide" {
            w262 = T5."Hidden" ("State")
            n101 = property class="VI"(reference=w268, error in=w267) -> (reference out=w265:refnum<vi>, error out=w266:errorcluster, "FP.State"=w264:T5)
            n102 = Not Equal?(x=w264, y=w262) -> (x != y?=w263:bool)
            n103 = case shown="True" w263 {
              tunnel: [w273 w274] -> w269
              tunnel: w266 -> [w272 w274]
              tunnel: w265 -> [w271 _]
              tunnel: w262 -> [w270 _]
              frame True {
                n104 = invoke class="VI" method="FP.Open"(reference=w271, error in=w272, "State"=w270) -> (error out=w273:errorcluster)  [unwired: 2 in, 4 out]
              }
              frame False {
              }
            }
          }
          frame "Minimize", "Minimized" {
            w275 = T5."Minimized" ("State")
            n105 = property class="VI"(reference=w281, error in=w280) -> (reference out=w278:refnum<vi>, error out=w279:errorcluster, "FP.State"=w277:T5)
            n106 = Not Equal?(x=w277, y=w275) -> (x != y?=w276:bool)
            n107 = case shown="True" w276 {
              tunnel: [w286 w287] -> w282
              tunnel: w279 -> [w285 w287]
              tunnel: w278 -> [w284 _]
              tunnel: w275 -> [w283 _]
              frame True {
                n108 = invoke class="VI" method="FP.Open"(reference=w284, error in=w285, "State"=w283) -> (error out=w286:errorcluster)  [unwired: 2 in, 4 out]
              }
              frame False {
              }
            }
          }
          frame "Maximize", "Maximized" {
            w288 = T5."Maximized" ("State")
            n109 = property class="VI"(reference=w294, error in=w293) -> (reference out=w291:refnum<vi>, error out=w292:errorcluster, "FP.State"=w290:T5)
            n110 = Not Equal?(x=w290, y=w288) -> (x != y?=w289:bool)
            n111 = case shown="True" w289 {
              tunnel: [w299 w300] -> w295
              tunnel: w292 -> [w298 w300]
              tunnel: w291 -> [w297 _]
              tunnel: w288 -> [w296 _]
              frame True {
                n112 = invoke class="VI" method="FP.Open"(reference=w297, error in=w298, "State"=w296) -> (error out=w299:errorcluster)  [unwired: 2 in, 4 out]
              }
              frame False {
              }
            }
          }
        }
        n113 = call <vilib>:"Add State(s) to Queue__jki_lib_state_machine.vi"("State(s) in (\"\")"=w235) -> ("States Out"=w234:string)  [unwired: 14 in]
      }
      frame "---------- Macro ----------" {
        # "Do not put any code in this frame.\n(It is a separator no-op. You can make a copy of this frame to create a new Macro frame)"
        n114 = call <vilib>:"Add State(s) to Queue__jki_lib_state_machine.vi"("State(s) in (\"\")"=w304) -> ("States Out"=w303:string)  [unwired: 14 in]
      }
      frame "Macro: Initialize" {
        w305 = "Data: Initialize\nInitialize Core Data\nUI: Initialize\nUI: Front Panel State >> Open\nData: Initialize Ring Map"  # Data: Initialize Initialize Core Data UI: Initialize UI: Front Panel State >> Open Data: Initialize Ring Map
        # "Initialization Macro\n(This is called once, when the VI starts)"
        n115 = call <vilib>:"Add State(s) to Queue__jki_lib_state_machine.vi"("State(s) in Front (\"\")"=w305, "State(s) in (\"\")"=w309) -> ("States Out"=w308:string)  [unwired: 13 in]
      }
      frame "Macro: Initialize Keys" {
        # "Do not put any code in this frame.\n(It is a separator no-op. You can make a copy of this frame to create a new Macro frame)"
        n116 = call <vilib>:"Add State(s) to Queue__jki_lib_state_machine.vi"("State(s) in Front (\"\")"="Actions: List Folder\nActions: Folder Subset\nData: Set Running Step >> 0\nActions: Read File\nData: Set Running Step >> -1\nActions: List Keys\nData: Update Rings" ("State(s) in Front (\"\")"), "State(s) in (\"\")"=w314) -> ("States Out"=w313:string)  [unwired: 13 in]
      }
      frame "Macro: Run Sequence" {
        # "File\nGraph"
        # "Do not put any code in this frame.\n(It is a separator no-op. You can make a copy of this frame to create a new Macro frame)"
        n117 = Unbundle By Name(w326) -> ("Files"=w325:path[], "Running Step"=w316:i32)
        n118 = Array Size(array=w325) -> (size(s)=w318:i32)
        n119 = Decrement(x=w318) -> (x-1=w317:i32)
        n120 = Less?(x=w316, y=w317) -> (x < y?=w315:bool)
        n121 = Increment(x=w316) -> (x+1=w323:i32)
        n122 = Format Into String(format string="Data: Set Running Step >> %1$d\nMacro: %2$s Sequence\nMacro: Run Sequence >> %2$s", w323, w319) -> (resulting string=w321:string)  [unwired: 2 in, 1 out]
        n123 = Select(t=w321, s=w315, f="Data: Set Running Step >> -1") -> (s? t:f=w320:string)
        n124 = call <vilib>:"Add State(s) to Queue__jki_lib_state_machine.vi"("State(s) in Front (\"\")"=w320, "State(s) in (\"\")"=w329) -> ("States Out"=w328:string)  [unwired: 13 in]
      }
      frame "Macro: Read Files" {
        # "Do not put any code in this frame.\n(It is a separator no-op. You can make a copy of this frame to create a new Macro frame)"
        n125 = call <vilib>:"Add State(s) to Queue__jki_lib_state_machine.vi"("State(s) in Front (\"\")"="Macro: Initialize Keys\nMacro: Run Sequence >> File" ("State(s) in Front (\"\")"), "State(s) in (\"\")"=w334) -> ("States Out"=w333:string)  [unwired: 13 in]
      }
      frame "Macro: File Sequence" {
        # "Do not put any code in this frame.\n(It is a separator no-op. You can make a copy of this frame to create a new Macro frame)"
        n126 = call <vilib>:"Add State(s) to Queue__jki_lib_state_machine.vi"("State(s) in Front (\"\")"="Actions: Read File" ("State(s) in Front (\"\")"), "State(s) in (\"\")"=w339) -> ("States Out"=w338:string)  [unwired: 13 in]
      }
      frame "Macro: Update Graphs" {
        # "Do not put any code in this frame.\n(It is a separator no-op. You can make a copy of this frame to create a new Macro frame)"
        n127 = call <vilib>:"Add State(s) to Queue__jki_lib_state_machine.vi"("State(s) in Front (\"\")"="Data: Initialize Graphs\nUI: Graph Labels\nMacro: Run Sequence >> Graph\nUI: Recolor Graphs" ("State(s) in Front (\"\")"), "State(s) in (\"\")"=w344) -> ("States Out"=w343:string)  [unwired: 13 in]
      }
      frame "Macro: Graph Sequence" {
        # "Do not put any code in this frame.\n(It is a separator no-op. You can make a copy of this frame to create a new Macro frame)"
        n128 = call <vilib>:"Add State(s) to Queue__jki_lib_state_machine.vi"("State(s) in Front (\"\")"="Actions: Extract Data\nUI: Update Graphs" ("State(s) in Front (\"\")"), "State(s) in (\"\")"=w349) -> ("States Out"=w348:string)  [unwired: 13 in]
      }
      frame "Macro: Exit" {
        # "Exit Macro\n(This is called once, when the VI exits)"
        n129 = Unbundle By Name(w356) -> ("Core.Close Panel on Exit?"=w355:bool)
        n130 = Select(t="UI: Front Panel State >> Close", s=w355, f="") -> (s? t:f=w352:string)
        n131 = call <vilib>:"Add State(s) to Queue__jki_lib_state_machine.vi"("State(s) in (\"\")"=w352, "State(s) at Back (\"\")"="Data: Cleanup\nExit") -> ("States Out"=w350:string)  [unwired: 13 in]
        n132 = call <vilib>:"Add State(s) to Queue__jki_lib_state_machine.vi"("State(s) in Front (\"\")"=w350, "State(s) in (\"\")"=w359) -> ("States Out"=w358:string)  [unwired: 13 in]
      }
      frame "---------- Actions ----------" {
        # "Template Separator\n(You can make a copy of, or modify, this frame)"
        n133 = call <vilib>:"Add State(s) to Queue__jki_lib_state_machine.vi"("State(s) in (\"\")"=w363) -> ("States Out"=w362:string)  [unwired: 14 in]
      }
      frame "Actions: List Folder" {
        # "Folder Index is a way to store the list of files in a particular folder.\nSpeeds up execution next time you want to list the folder."
        # "if path = folder, return list of files according to filter.\notherwise return file name"
        # "List Folder.\n(List folder contents)"
        n134 = case shown="\"TDMS\"" "Data Type" {
          tunnel: ["*.itx" ("pattern") "*.dat" ("pattern") "*.tdms" ("pattern")] -> w364
          tunnel: "DAT header length" -> [_ w380 _]
          tunnel: [0 ("DAT header length") w380 0 ("DAT header length")] -> w365
          frame Default {
          }
          frame "DAT" {
          }
          frame "TDMS" {
          }
        }
        "pattern" <- w364
        n135 = case shown="False" "Use Folder Index File?" {
          tunnel: [w389 w410] -> w368
          tunnel: "File or Folder Path" -> [w391 w411]
          tunnel: "Generate Folder Index File?" -> [w384 _]
          tunnel: w364 -> [w388 _]
          tunnel: w369 -> [w387 w409]
          tunnel: [w385 w408] -> w370
          frame False {
            n136 = File/Directory Info(path=w391, error in=w387) -> (directory=w390:bool, error out=w386:errorcluster)  [unwired: 5 out]
            n137 = case shown="True" w390 {
              tunnel: [w394 w402] -> w389
              tunnel: w391 -> [w393 w396]
              tunnel: w384 -> [_ w395]
              tunnel: w388 -> [_ w401]
              tunnel: w386 -> [w392 w399]
              tunnel: [w392 w400] -> w385
              frame False {
                n138 = Build Array(w393) -> (w394:path[])
              }
              frame True {
                n139 = call <vilib>:"Recursive File List.vi"("pattern"=w401, "error in (no error)"=w399, "Folder Path"=w396) -> ("error out"=w398:errorcluster, "All Files in Dir"=w402:path[], "dup Folder Path"=w397:path)  [unwired: 4 in, 2 out]
                n140 = case shown="False" w395 {
                  tunnel: w402 -> [_ w407]
                  tunnel: w397 -> [_ w406]
                  tunnel: w398 -> [w403 w405]
                  tunnel: [w403 w404] -> w400
                  frame False {
                  }
                  frame True {
                    n141 = call "Create Folder Index.vi"("error in (no error)"=w405, "File or Folder Path"=w406, "All Files in Dir"=w407) -> ("error out"=w404:errorcluster)  [unwired: 8 in]
                  }
                }
              }
            }
          }
          frame True {
            n142 = call "Read Folder Index.vi"("error in (no error)"=w409, "File or Folder Path"=w411) -> ("error out"=w408:errorcluster, "Files"=w410:path[])  [unwired: 8 in]
          }
        }
        n143 = Bundle By Name(cluster=w366, "Files"=w368, "Append Index"=w365) -> (w367:T9)
        n144 = call <vilib>:"Add State(s) to Queue__jki_lib_state_machine.vi"("State(s) in (\"\")"=w377) -> ("States Out"=w376:string)  [unwired: 14 in]
      }
      frame "Actions: Folder Subset" {
        # "Action: Folder Subset.\n2. Subset of files)"
        n145 = Unbundle By Name(w419) -> ("Files"=w421:path[])
        n146 = Less Than 0?(x="offset") -> (x < 0?=w414:bool)
        n147 = Less Than 0?(x="length") -> (x < 0?=w413:bool)
        n148 = Or(x=w414, y=w413) -> (x .or. y?=w412:bool)
        n149 = case shown="False" w412 {
          tunnel: w421 -> [w428 w429]
          tunnel: [w425 w429] -> w418
          tunnel: "length" -> [w427 _]
          tunnel: "offset" -> [w426 _]
          frame False {
            n150 = Array Subset(array=w428, index=w426, length=w427) -> (w425:path[])
          }
          frame True {
          }
        }
        n151 = for {
          tunnel: w418 -> [w431] mode=indexing
          tunnel: [w430] -> w417 mode=indexing
          n152 = File/Directory Info(path=w431) -> (last mod=w432:timestamp)  [unwired: 1 in, 6 out]
          n153 = Get Date/Time String(seconds (now)=w432) -> (date string=w434:string, time string=w433:string)  [unwired: 2 in]
          n154 = Build Array(w434, w433) -> (w430:string[])
        }
        "time" <- w417
        n155 = Bundle By Name(cluster=w419, "Files"=w418) -> (w420:T9)
        n156 = call <vilib>:"Add State(s) to Queue__jki_lib_state_machine.vi"("State(s) in (\"\")"=w424) -> ("States Out"=w423:string)  [unwired: 14 in]
      }
      frame "Actions: List Keys" {
        # "Template Separator\n(You can make a copy of, or modify, this frame)"
        n157 = Unbundle By Name(w439) -> ("Data Map"=w444:T7[])
        n158 = Index Array(array=w444) -> (element=w443:T7)  [unwired: 1 in]
        n159 = call "List Map Keys and Values.vim"("error in (no error)"=w441, "map in"=w443) -> ("error out"=w442:errorcluster, "Keys"=w435:string[])  [unwired: 6 in, 2 out]
        n160 = for {
          tunnel: w435 -> [_] mode=indexing
          tunnel: [w447] -> w436 mode=indexing
          i -> [w448]
          n161 = Number To Decimal String(number=w448) -> (decimal integer string=w447:string)  [unwired: 1 in]
        }
        n162 = Bundle By Name(cluster=w439, "Wavenames"=w435) -> (w440:T9)
        n163 = Build Array(w436, w435) -> (w438:string[][])
        n164 = Transpose 2D Array(2D array=w438) -> (transposed array=→"Index, Wavenames":string[][])
        n165 = call <vilib>:"Add State(s) to Queue__jki_lib_state_machine.vi"("State(s) in (\"\")"=w446) -> ("States Out"=w445:string)  [unwired: 14 in]
      }
      frame "Actions: Read File" {
        # "Template Separator\n(You can make a copy of, or modify, this frame)"
        n166 = Unbundle By Name(w454) -> ("Data Map"=w449:T7[], "Files"=w463:path[], "Running Step"=w452:i32, "Append Index"=w460:i32)
        n167 = Index Array(array=w463, index=w452) -> (element=w462:path)
        n168 = call "Data Read.vi"("Append Index"=w460, "error in (no error)"=w461, "path"=w462) -> ("error out"=w457:errorcluster, "Notes"=→"Notes":string, "Data (Dictionary)"=w458:T11[])  [unwired: 5 in, 1 out]
        n169 = call "Convert Dictionary to Map.vim"("error in (no error)"=w457, "Data (Dictionary)"=w458) -> ("error out"=w456:errorcluster, "map out"=w450:T7)  [unwired: 8 in]
        n170 = Empty Array?(array=w449) -> (empty?=w451:bool)
        n171 = case shown="True" w451 {
          tunnel: [w467 w470] -> w453
          tunnel: w449 -> [w468 _]
          tunnel: w450 -> [w466 w469]
          frame False {
            n172 = Build Array (concatenate)(w468, w466) -> (w467:T7[])
          }
          frame True {
            n173 = Build Array(w469) -> (w470:T7[])
          }
        }
        n174 = Bundle By Name(cluster=w454, "Data Map"=w453) -> (w455:T9)
        n175 = call <vilib>:"Add State(s) to Queue__jki_lib_state_machine.vi"("State(s) in (\"\")"=w465) -> ("States Out"=w464:string)  [unwired: 14 in]
      }
      frame "Actions: Extract Data" {
        # "Template Separator\n(You can make a copy of, or modify, this frame)"
        n176 = Unbundle By Name(w471) -> ("A vs B"=w482:cluster{dbl[], dbl[]}[], "C vs D"=w478:cluster{dbl[], dbl[]}[], "E"=w474:dbl[][])
        n177 = Unbundle By Name(w471) -> ("Data Map"=w496:T7[], "Running Step"=w483:i32, "ring map"=w484:map{string, refnum<vi>})
        n178 = for {
          tunnel: w496 -> [w509]
          tunnel: w484 -> [w513]
          tunnel: string[] ["B", "A", "D", "C", "E", "N1", "N2", "N3", "N4", "N5"] ("key") -> [w514] mode=indexing
          tunnel: [w512] -> w480 mode=indexing
          tunnel: w483 -> [w508]
          # "each"
          n179 = Look In Map(map=w513, key=w514) -> (value=w516:refnum<vi>)  [unwired: 1 in, 1 out]
          n180 = property class="Ring"(reference=w516) -> ("RingText.Text"=w515:string)  [unwired: 1 in, 2 out]
          n181 = Index Array(array=w509, index=w508) -> (element=w507:T7)
          n182 = Look In Map(map=w507, key=w515) -> (value=w511:variant)  [unwired: 1 in, 1 out]
          n183 = Variant To Data(type=dbl[] [], Variant=w511) -> (data=w512:dbl[])  [unwired: 1 in, 1 out]
        }
        n184 = Index Array(array=w480) -> (element #1=w494:dbl[], element #2=w493:dbl[], element #3=w492:dbl[], element #4=w491:dbl[], element #5=w473:dbl[], element #6=w490:dbl[], element #7=w489:dbl[], element #8=w488:dbl[], element #9=w487:dbl[], element #10=w486:dbl[])  [unwired: 20 in]
        n185 = Bundle(w494, w493) -> (w481:cluster{dbl[], dbl[]})  [unwired: 1 in]
        n186 = Bundle(w492, w491) -> (w476:cluster{dbl[], dbl[]})  [unwired: 1 in]
        n187 = Build Array (concatenate)(w482, w481) -> (w479:cluster{dbl[], dbl[]}[])
        n188 = Build Array (concatenate)(w478, w476) -> (w477:cluster{dbl[], dbl[]}[])
        n189 = Build Array (concatenate)(w474, w473) -> (w475:dbl[][])
        n190 = for {
          tunnel: w490 -> [w505] mode=indexing
          tunnel: w489 -> [w504] mode=indexing
          tunnel: w488 -> [w503] mode=indexing
          tunnel: w487 -> [w502] mode=indexing
          tunnel: w486 -> [w501] mode=indexing
          tunnel: [w506] -> w485 mode=indexing
          n191 = Bundle By Name(cluster=T8 {"N1"=0.0, "N2"=0.0, "N3"=0.0, "N4"=0.0, "N5"=0.0} ("N"), "N1"=w505, "N2"=w504, "N3"=w503, "N4"=w502, "N5"=w501) -> (w506:T8)
        }
        "N" <- w485
        n192 = Bundle By Name(cluster=w471, "A vs B"=w479, "C vs D"=w477, "E"=w475) -> (w472:T9)
        n193 = call <vilib>:"Add State(s) to Queue__jki_lib_state_machine.vi"("State(s) in (\"\")"=w499) -> ("States Out"=w498:string)  [unwired: 14 in]
      }
      frame "---------- Graph ----------" {
        # "Template Separator\n(You can make a copy of, or modify, this frame)"
        n194 = call <vilib>:"Add State(s) to Queue__jki_lib_state_machine.vi"("State(s) in (\"\")"=w520) -> ("States Out"=w519:string)  [unwired: 14 in]
      }
    }
  }
